vi "Configure Measurement Threshold.vi"(7 "Low Reference (10.0)":dbl=10.0, 8 "error in (no error)":errorcluster, 9 "High Reference (90.0)":dbl=90.0, 10 "Mid Reference (50.0)":dbl=50.0, 11 "VISA resource name":refnum<visa-resource-name>) -> (0 "error out":errorcluster, 3 "VISA resource name out":refnum<visa-resource-name>)   [LabVIEW 2017, in "Agilent 6000 Series.lvlib"]
doc: "This VI configures the reference levels in percents for waveform measurements. \n\nYou must call this VI before you call the ag6000 Read Waveform Measurement.vi or ag6000 Fetch Waveform Measurement.vi to take a rise time, fall time, width negative, width positive, duty cycle negative, or duty cycle positive measurement."
uses:
  <instrlib>/Agilent 6000 Series/Agilent 6000 Series.lvlib
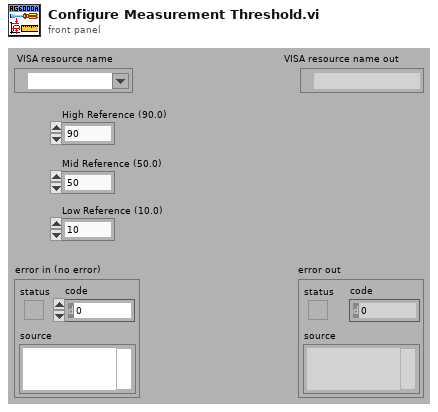
[diagram p1: front panel]
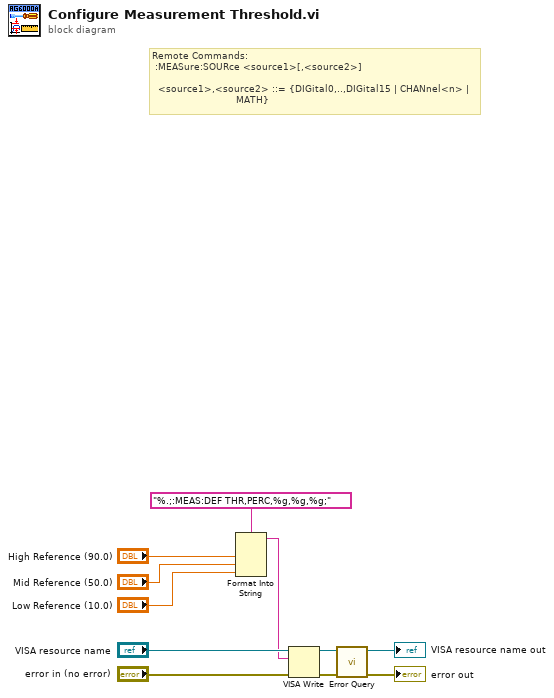
[diagram p0: block diagram]
diagram:
  # "Remote Commands:\n :MEASure:SOURce <source1>[,<source2>]\n\n  <source1>,<source2> ::= {DIGital0,..,DIGital15 | CHANnel<n> | \n                            MATH}"
  n1 = Format Into String(format string="%.;:MEAS:DEF THR,PERC,%g,%g,%g;", "High Reference (90.0)", "Mid Reference (50.0)", "Low Reference (10.0)") -> (resulting string=w4:string)  [unwired: 2 in, 1 out]
  n2 = VISA Write(VISA resource name="VISA resource name", write buffer=w4, error in (no error)="error in (no error)") -> (VISA resource name out=w7:refnum<visa-resource-name>, error out=w6:errorcluster)  [unwired: 1 out]
  n3 = call <instrlib>:"Error Query.vi"("error in (no error)"=w6, "VISA resource name"=w7) -> ("error out"=→"error out":errorcluster, "VISA resource name out"=→"VISA resource name out":refnum<visa-resource-name>)  [unwired: 6 in, 2 out]
